vi "Dashboard Main.vi"() -> ()   [LabVIEW 2015]
uses:
  <vilib>/Utility/miscctls.llb/LVRowAndColumnTypeDef.ctl
  <vilib>/event_ctls.llb/eventvkey.ctl
  <vilib>/Rock Robotics/WPI/Dashboard/WPI_DashboardLogging Global.vi
  <vilib>/Rock Robotics/Network Tables/NT Write Boolean.vi
  <vilib>/Rock Robotics/Network Tables/NT Read Boolean.vi
  <vilib>/Utility/config.llb/Write Key (String).vi
  <vilib>/Utility/config.llb/Write Key (I32).vi
  <vilib>/Utility/config.llb/NI_LVConfig.lvlib
  <vilib>/vision/NI_Vision_Development_Module.lvlib
panel:
  out "Best Box":dbl[](array[numeric])
  in  "TCP":refnum<k5>
  in  "Rec Mode":enum32{"Stop", "Record", "Playback"}(radio)
  in  "Vision":u16(ring) items=["Camera Off", "USB Camera SW", "USB Camera HW", "IP Camera"]
  out "Camera IP":string
  out "Image Message":string="Timeout in Camera Communications"
  in  "Dashboard Tab":T1(tab)
  out "R Abv 60000":bool
  out "L Abv 60000":bool
  out "On Goal":bool
  out "Angler":dbl
  out "Right Shooter":dbl
  out "Left Shooter":dbl
  out "Right Ready":bool
  out "Left Ready":bool
  out "NT Connection":bool
  in  "Camera Settings":T2={"Frame Rate"=30, "Compression"=30, "Size"=1} {"Frame Rate" scale=1.0..30.0; "Size" items=["640x480", "320x240", "160x120"]}
  out "Gyro":cluster{dbl, dbl}(knob) scale=0.0..360.0
  out "Mode":T3(ring)=enum."Auto Disabled"
  in  "DB Camera Config":bool
  out "fps":dbl format="%#.1g"
  out "Mbps":dbl format="%#.1g"
  out "Mbps LED":bool
  out "View":bool
  in  "DB/String 9":string
  in  "DB/String 8":string
  in  "DB/String 7":string
  in  "DB/String 6":string
  in  "DB/String 5":string
  in  "DB/String 4":string
  in  "DB/String 3":string
  in  "DB/String 2":string
  in  "DB/String 1":string
  in  "DB/String 0":string
  in  "DB/Slider 0":dbl(slide) scale=0.0..5.0
  in  "DB/Slider 1":dbl(slide) scale=0.0..5.0
  in  "DB/Slider 2":dbl(slide) scale=0.0..5.0
  in  "DB/Slider 3":dbl(slide) scale=0.0..5.0
  out "DB/LED 3":bool
  out "DB/LED 2":bool
  out "DB/LED 1":bool
  out "DB/LED 0":bool
  in  "DB/Button 3":bool
  in  "DB/Button 2":bool
  in  "DB/Button 1":bool
  in  "DB/Button 0":bool caption="New Name"
  in  "Debug Camera":bool
  in  "Starting Direction":enum32{"Radio Selection 1", "Radio Selection 2"}(radio)
  in  "Defense to Cross":u16(ring) items=["Low Bar", "Moat", "Ramparts", "Rock Wall", "Rough Terrain", "Cheval", "Portculis"]
  in  "Starting Position":u16(ring) items=["1", "2", "3", "4", "5", "Spy"]
  in  "Autonomous Mode":u16(ring) items=["Do Nothing", "Drive to OW", "Drive through OW", "Shoot"]
  in  "Test Slider":dbl(slide) scale=0.0..100.0 scale format="%#_3g"
  in  "On/Off":bool caption="Solenoid"
  in  "Test Name":u16(ring) items=["Select the test to run..."]
  in  "Test Tree":string(tree)
  in  "Motor":cluster{"Value":dbl, "Enable":bool} {"Value" scale=-1.0..1.0 scale format="%#_3g"}
  out "Progress":T4 {"Test Progress" scale=0.0..100.0}
  in  "Rev/Fwd":cluster{"Forward":bool, "Reverse":bool}
  in  "Test Ring":u16(ring) items=["Monochrome", "Color"]
  out "Cmd Status":string
  in  "Execute Command":bool
  in  "Command Params":string[][](table)
  in  "Command Selection":i32(listbox)
  in  "CheckList":i32(listbox)
  out "Tree":string(tree)
  out "Camera Image":T5(plugin-control)
  out "Background":bool
  in  "Select Auto":string(combo)
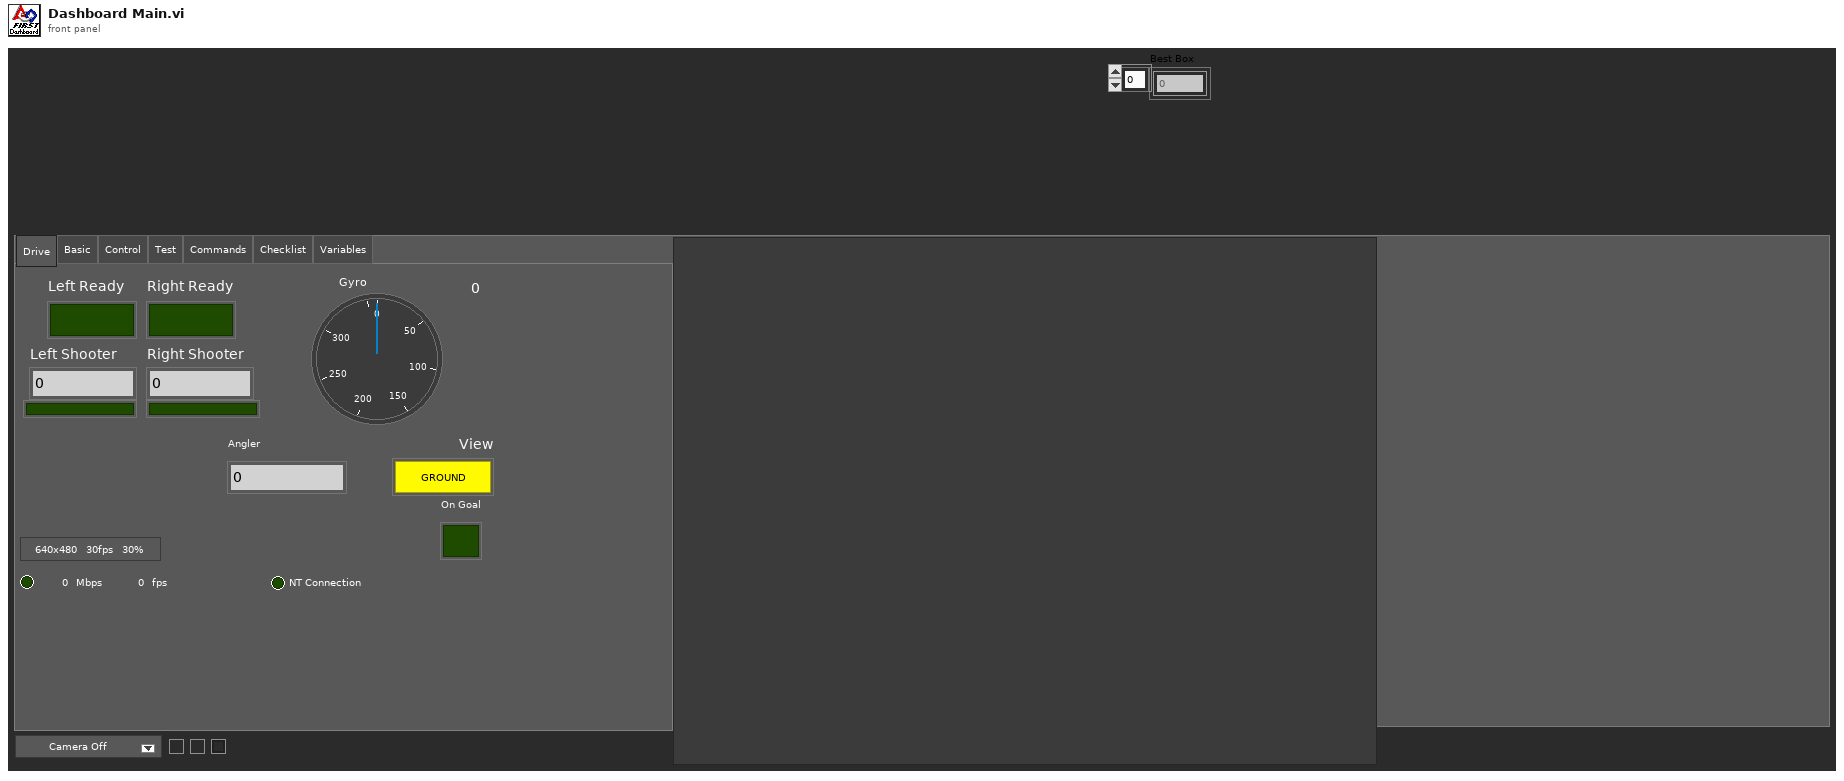
[diagram p1: front panel]
types:
  T1 = enum32{"Drive", "Basic", "Control", "Test", "Commands", "Checklist", "Variables"}
  T2 = cluster{"Frame Rate":i32, "Compression":i32, "Size":u16}
  T3 = enum8{"Tele-Op Disabled", "Tele-Op Enabled", "Auto Disabled", "Auto Enabled", "Test Disabled", "Test Enabled", "Disconnected", "No Code", "E-Stop"}
  T4 = cluster{"Test Progress":u8, "Test Progress Text":string}
  T5 = typedef "IMAQ Image.ctl" = refnum<image>
  T6 = cluster{"IDs":cluster{"RPC field ID":u16, "Unique ID":u16}, "String":string}
  T7 = enum32{"Drive", "Basic", "Custom", "Test", "Checklist", "Variables"}
  T8 = typedef "Image Type" = u32
  T9 = cluster{"Camera Image":refnum<vi>, "Dashboard Tab":refnum<vi>, "Background":refnum<vi>, "Vision":refnum<vi>, "Rec Mode":refnum<vi>, "Test Slider":refnum<vi>, "On/Off ":refnum<vi>, "Test Ring":refnum<vi>, "Rev/Fwd":refnum<vi>, "Test Name":refnum<vi>, "Motor":refnum<vi>, "Progress":refnum<vi>, "CheckList":refnum<vi>, "Tree":refnum<vi>, "Test Tree":refnum<vi>, "Command Params":refnum<vi>, "Command Selection":refnum<vi>, "Execute Command":refnum<vi>, "Cmd Status":refnum<vi>}
  T10 = cluster{"Error Strings":string, "Disable Counts":cluster{u16, u16}, "Rail Faults":cluster{u16, u16, u16}, "Robot IP":string, "DB Mode":u8, "Event Info":cluster{"Name":string, "Type":u8, "Number":u16, "Replay":u8}, "Camera Addr":string}
  T11 = cluster{"Storage":cluster{"Disk Free":u64, "RAM Block":u32, "RAM free":u32}, "CPU Utilization":cluster{"CPU % ISR":sgl, "CPU % Time Crit":sgl, "CPU % Timed Str":sgl, "CPU % High":sgl, "CPU % Above":sgl, "CPU % Normal":sgl, "CPU % Low":sgl}, "CAN":cluster{"% Bus Utilization":sgl, "Bus Off Cnt":u32, "TX_FIFO Full Cnt":u32, "Receive Error Cnt":u8, "Transmit Error Cnt":u8}, "HID":cluster{"HID Outputs":u32, "Rumble Low":u16, "Rumble High":u16}[]}
  T12 = cluster{"Status bits":cluster{"Test Mode":bool, "Autonomous":bool, "Enabled":bool, "Code Start":bool, "Brownout":bool, "Reserved 2":bool, "Reserved 3":bool, "E-Stop":bool}, "Code Trace":cluster{"Disabled":bool, "TeleOp":bool, "Auto":bool, "Test":bool}, "Controller Type":enum16{"unknown", "cRIO", "roboRio"}, "Code?":enum16{"unknown", "noCode", "code"}, "Battery V":dbl}
  T13 = cluster{"Control Bits":cluster{"TestMode":bool, "Autonomous":bool, "Enabled":bool, "FMS Present":bool, bool, bool, bool, "E-Stop":bool}, "Team Station ":u8, "Countdown":sgl, "Joystick Values":cluster{"Axes":dbl[], "Buttons":bool[], "POVs":i16[]}[]}
  T14 = typedef "NI_LVConfig.lvlib/Config Data RefNum.ctl" = refnum<k1>
  T15 = cluster{"Operation":enum16{"Update", "Clear"}, "Color Box":u32}[]
  T16 = typedef "eventvkey.ctl" = enum16{"ASCII", "Enter", "Return", "Shift", "Ctrl", "Alt", "Cmd", "Opt", "Caps", "NumLock", "Clear", "Break", "Up", "Down", "Left", "Right", "Insert", "Delete", "Home", "End", "PageUp", "PageDown", "Escape", "Help", "Pause", "ScrollLock", "F1", "F2", "F3", "F4", "F5", "F6", "F7", "F8", "F9", "F10", "F11", "F12", "F13", "F14", "F15", "F16", "F17", "F18", "F19", "F20", "F21", "F22", "F23", "F24", "Play", "VolumeUp", "VolumeDown", "Mute", "Two Byte Char"}
  T17 = cluster{"Image Size":bool, "Image Type":bool, "Pixel Value":bool, "ROI Information":bool, "Zoom Factor":bool}
  T18 = enum8{"Enabled", "Disabled", "Disabled and Grayed Out"}
  T19 = cluster{"Operation":enum16{"Update", "Clear"}, "Color Box":u32}
  T20 = typedef "LVRowAndColumnTypeDef.ctl" = cluster{"Row":i32, "Column":i32}
  T21 = cluster{"Shift":bool, "Ctrl":bool, "Alt":bool, "Cmd":bool, "Opt":bool}
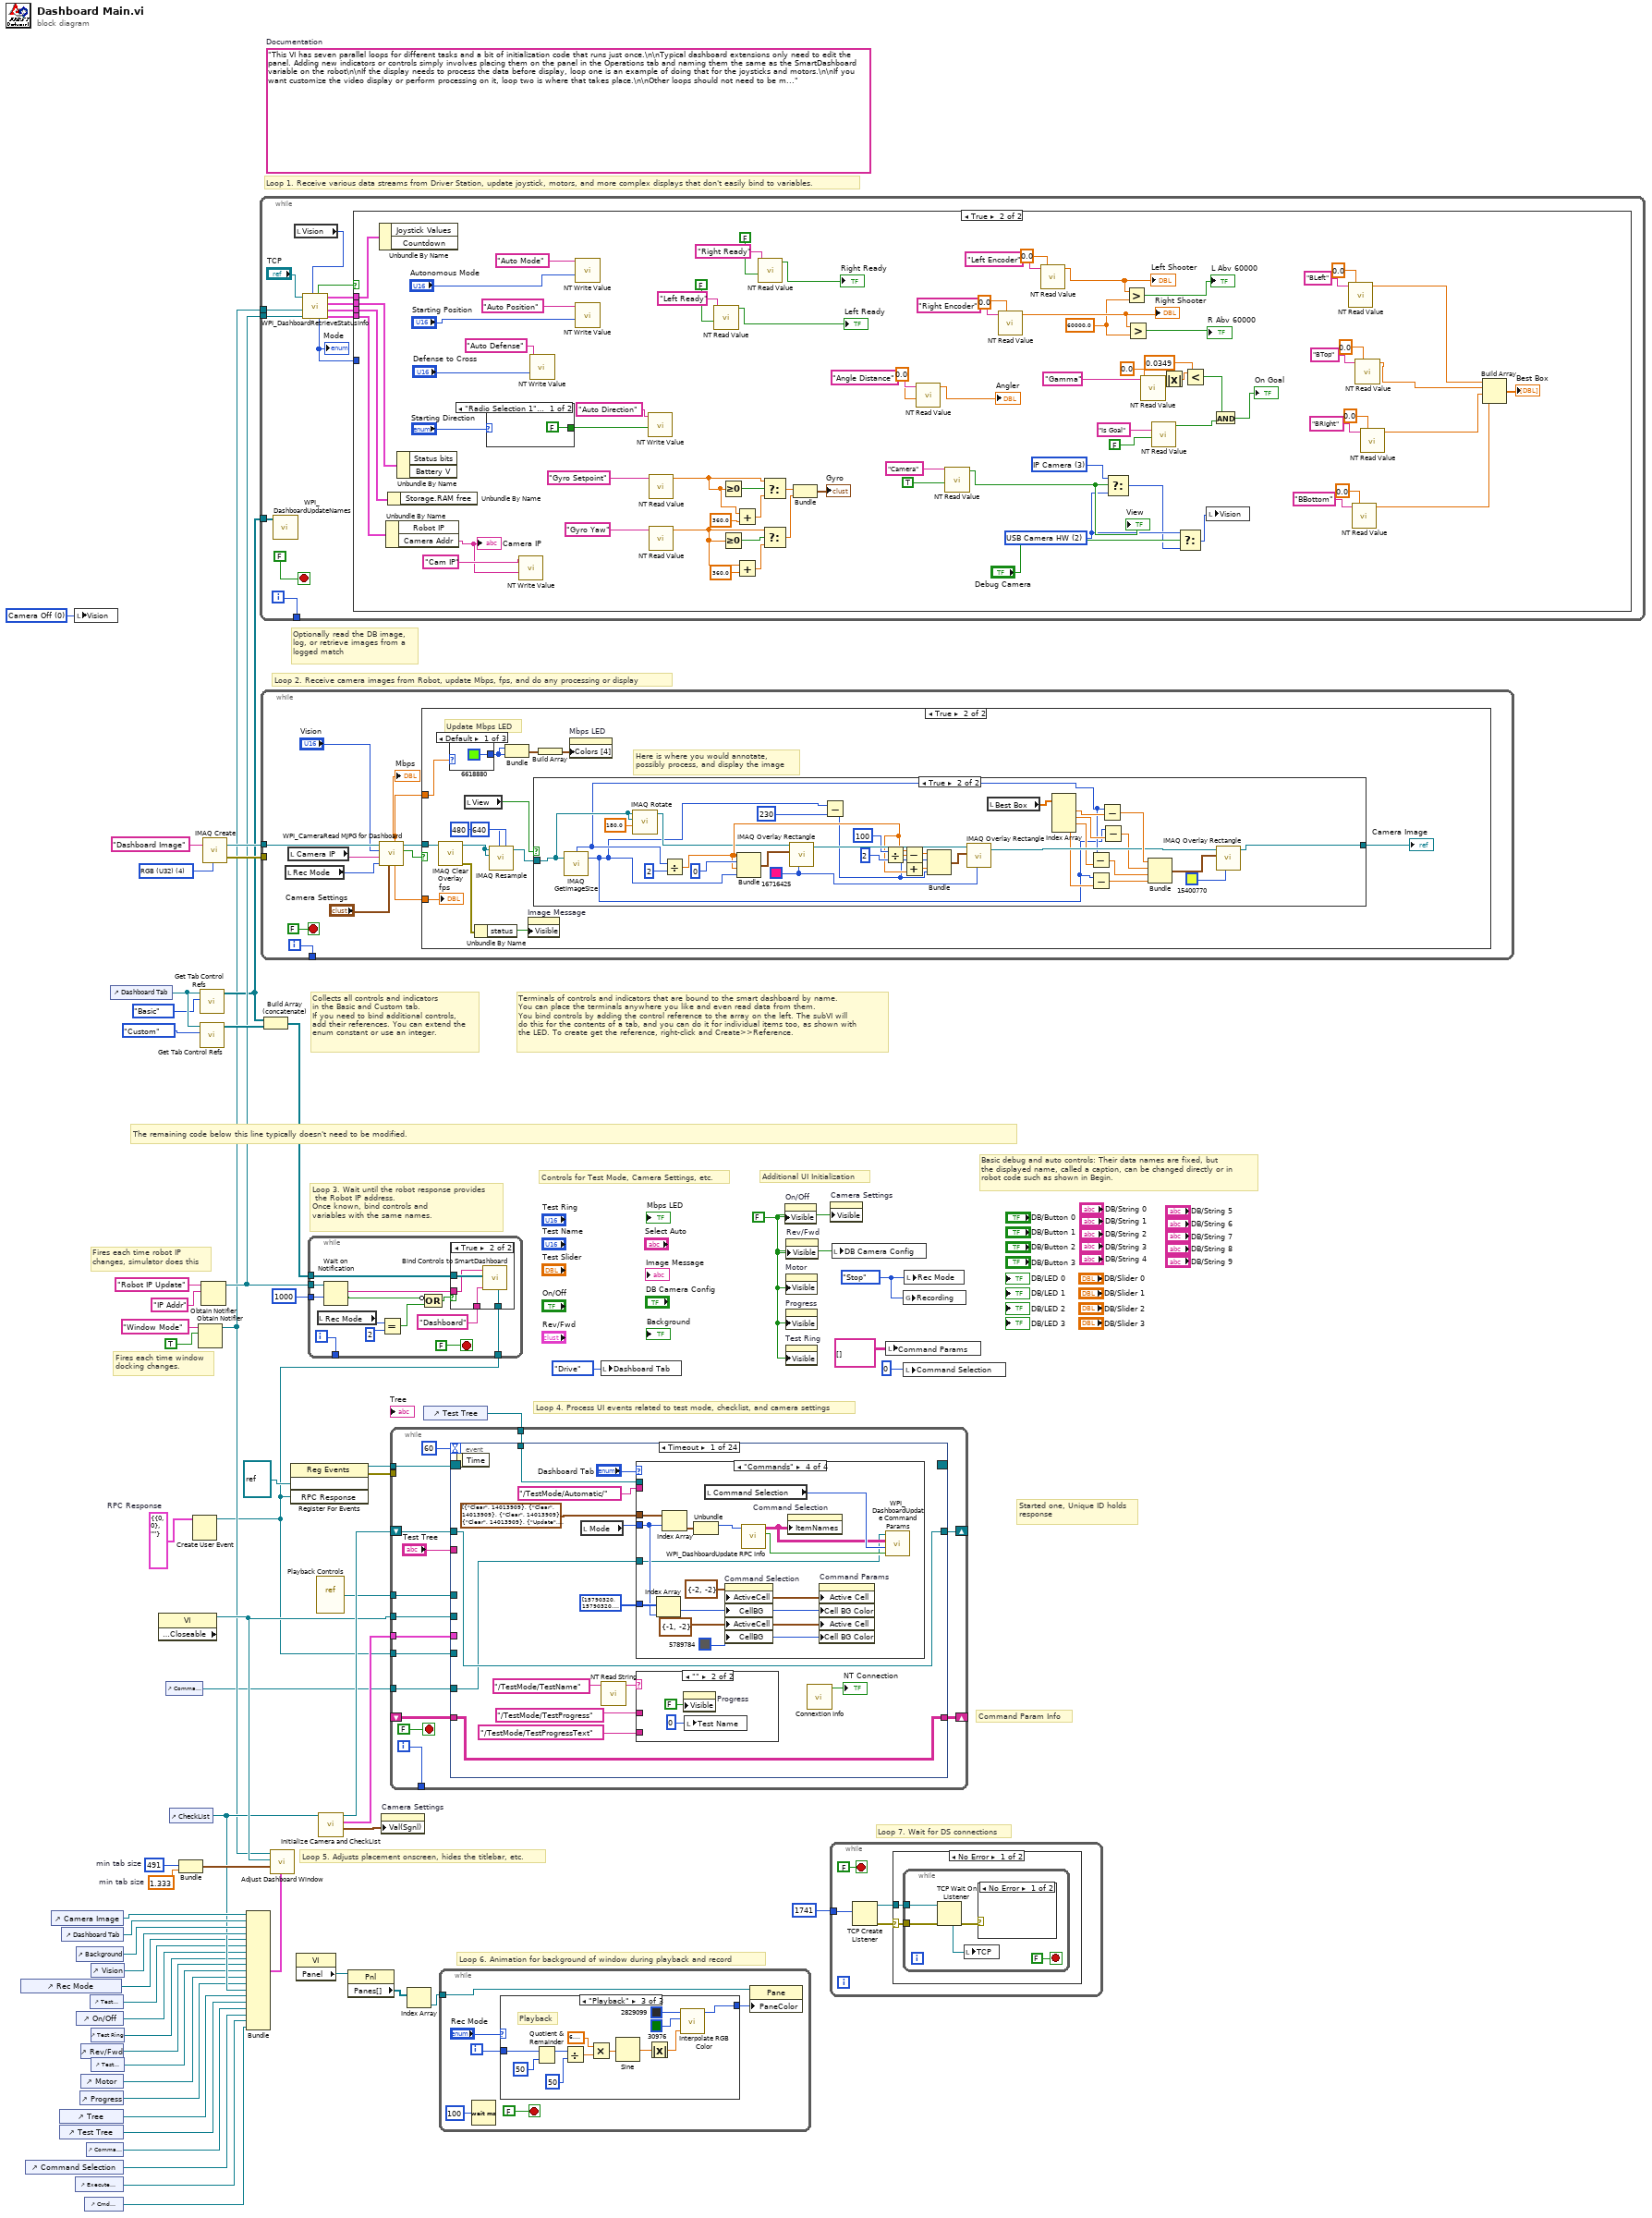
[diagram p0: block diagram]
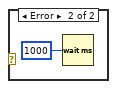
[diagram p2: hidden frame]
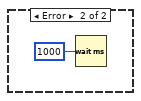
[diagram p3: hidden frame]
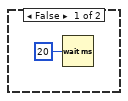
[diagram p4: hidden frame]
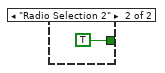
[diagram p5: hidden frame]
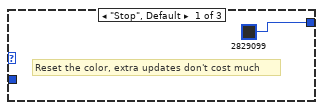
[diagram p6: hidden frame]
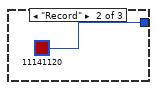
[diagram p7: hidden frame]
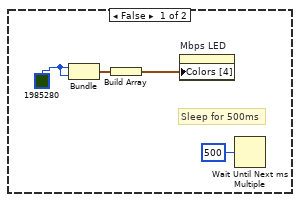
[diagram p9: hidden frame]
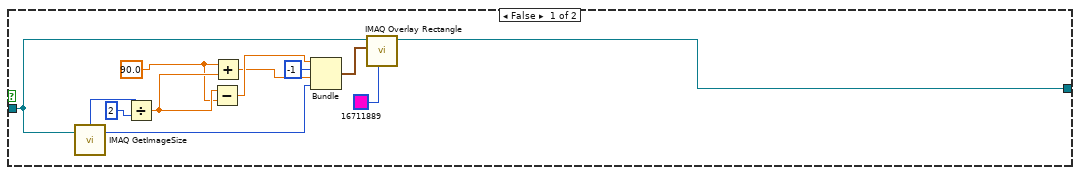
[diagram p10: hidden frame]
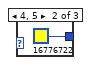
[diagram p11: hidden frame]
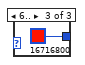
[diagram p12: hidden frame]
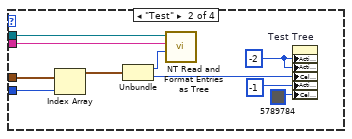
[diagram p14: hidden frame]
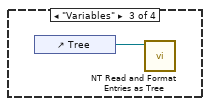
[diagram p15: hidden frame]
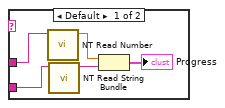
[diagram p16: hidden frame]
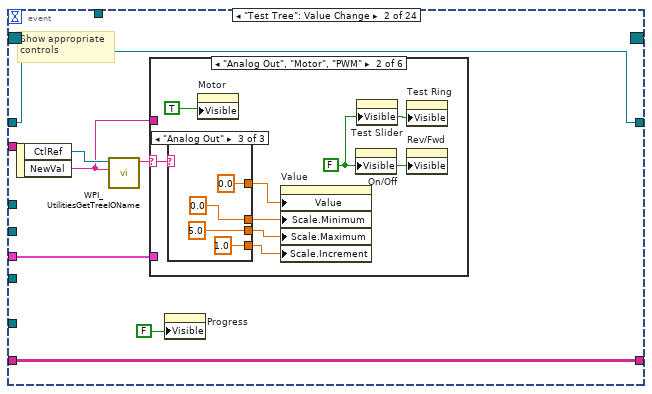
[diagram p17: hidden frame]
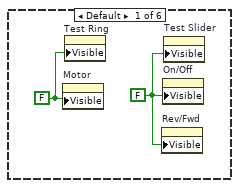
[diagram p18: hidden frame]
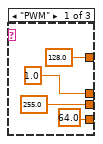
[diagram p19: hidden frame]
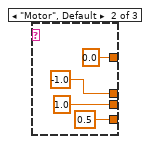
[diagram p20: hidden frame]
diagram:
  w1 = u16 0 items=["Camera Off", "USB Camera SW", "USB Camera HW", "IP Camera"] ("Vision")
  w9 = T6 {"IDs"={"RPC field ID"=0, "Unique ID"=0}, "String"=""}  # RPC Response
  w34 = 491  # min tab size
  w33 = 1.333  # min tab size
  w42 = enum32{"Stop", "Record", "Playback"}."Stop" ("Rec Mode")
  w16 = FALSE ("Visible")
  (unwired) "This VI has seven parallel loops for different tasks and a bit of initialization code that runs just once.\n\nTypical dashboard extensions only need to edit the panel. Adding new indicators or controls simply involves placing them on the panel in the Operations tab and naming them the same as the SmartDashboard variable on the robot\n\nIf the display needs to process the data before display, loop one is an example of doing that for the joysticks and motors.\n\nIf you want customize the video display or perform processing on it, loop two is where that takes place.\n\nOther loops should not need to be modified. They are pretty standard, and document the task they perform."  # Documentation
  w62 = T8 4 items=["Grayscale (U8)", "Grayscale (I16)", "Grayscale (SGL)", "Complex (CSG)", "RGB (U32)", "HSL (U32)", "RGB (U64)"] ("Image Type")
  # "Optionally read the DB image,\nlog, or retrieve images from a\nlogged match"
  # "Command Param Info"
  # "Started one, Unique ID holds\nresponse"
  # "Loop 7. Wait for DS connections"
  # "Basic debug and auto controls: Their data names are fixed, but\nthe displayed name, called a caption, can be changed directly or in\nrobot code such as shown in Begin."
  # "Controls for Test Mode, Camera Settings, etc."
  # "Additional UI Initialization"
  # "Loop 6. Animation for background of window during playback and record"
  # "Fires each time robot IP\nchanges, simulator does this"
  # "Fires each time window\ndocking changes."
  # "Collects all controls and indicators\nin the Basic and Custom tab.\nIf you need to bind additional controls,\nadd their references. You can extend the\nenum constant or use an integer."
  # "The remaining code below this line typically doesn't need to be modified."
  # "Loop 4. Process UI events related to test mode, checklist, and camera settings"
  # "Terminals of controls and indicators that are bound to the smart dashboard by name.\nYou can place the terminals anywhere you like and even read data from them.\nYou bind controls by adding the control reference to the array on the left. The subVI will\ndo this for the contents of a tab, and you can do it for individual items too, as shown with\nthe LED. To create get the reference, right-click and Create>>Reference."
  # "Loop 3. Wait until the robot response provides\n the Robot IP address.\nOnce known, bind controls and\nvariables with the same names."
  # "Loop 5. Adjusts placement onscreen, hides the titlebar, etc."
  # "Loop 1. Receive various data streams from Driver Station, update joystick, motors, and more complex displays that don't easily bind to variables."
  # "Loop 2. Receive camera images from Robot, update Mbps, fps, and do any processing or display"
  n1 = control-ref of="Rec Mode"() -> (w22:refnum<vi>)
  n2 = control-ref of="Command Selection"() -> (w8:refnum<vi>)
  n3 = control-ref of="Camera Image"() -> (w37:refnum<vi>)
  n4 = control-ref of="Tree"() -> (w26:refnum<vi>)
  n5 = control-ref of="Test Tree"() -> (w25:refnum<vi>)
  n6 = control-ref of="Dashboard Tab"() -> (w36:refnum<vi>)
  n7 = local write "Vision"(w1) -> ()
  n8 = control-ref of="Execute Command"() -> (w10:refnum<vi>)
  n9 = control-ref of="Background"() -> (w31:refnum<vi>)
  n10 = control-ref of="On/Off"() -> (w20:refnum<vi>)
  n11 = control-ref of="Progress"() -> (w17:refnum<vi>)
  n12 = control-ref of="Rev/Fwd"() -> (w18:refnum<vi>)
  n13 = control-ref of="Motor"() -> (w23:refnum<vi>)
  n14 = control-ref of="Cmd Status"() -> (w4:refnum<vi>)
  n15 = control-ref of="Command Params"() -> (w11:refnum<vi>)
  n16 = control-ref of="Test Slider"() -> (w21:refnum<vi>)
  n17 = control-ref of="Vision"() -> (w35:refnum<vi>)
  n18 = control-ref of="Test Ring"() -> (w19:refnum<vi>)
  n19 = control-ref of="Test Name"() -> (w24:refnum<vi>)
  n20 = control-ref of="Dashboard Tab"() -> (w40:refnum<vi>)
  n21 = property class="VI" props=["Front Panel.Closeable"]() -> (reference out=w41:refnum<vi>)  [unwired: 2 in, 2 out]
  n22 = control-ref of="Command Params"() -> (w3:refnum<vi>)
  n23 = control-ref of="CheckList"() -> (w27:refnum<vi>)
  n24 = Bundle("min tab size"=w34, "min tab size"=w33) -> (w32:cluster{"min tab size":i32, "min tab size":dbl})  [unwired: 1 in]
  n25 = Create User Event(user event datatype=w9) -> (user event=w5:refnum<user-event>)  [unwired: 1 in, 1 out]
  n26 = Obtain Notifier(name (unnamed)="Window Mode", notification data type=TRUE) -> (notifier out=w13:refnum<notifier>)  [unwired: 2 in, 2 out]
  n27 = call <vilib>:"Get Tab Control Refs.vi"("Page Index"=T7."Basic" ("Dashboard Tab"), "TabControl in"=w40) -> ("ControlsOnPage"=w14:refnum<vi>[])  [unwired: 9 in]
  n28 = call <vilib>:"Get Tab Control Refs.vi"("Page Index"=T7."Custom" ("Dashboard Tab"), "TabControl in"=w40) -> ("ControlsOnPage"=w39:refnum<vi>[])  [unwired: 9 in]
  n29 = Obtain Notifier(name (unnamed)="Robot IP Update", notification data type="IP Addr" ("name (unnamed)")) -> (notifier out=w15:refnum<notifier>)  [unwired: 2 in, 2 out]
  n30 = call "IMAQ Create"("Image Name"="Dashboard Image", "Image Type"=w62) -> ("New Image"=w60:T5, "error out"=w59:errorcluster)  [unwired: 2 in, 1 out]
  n31 = Bundle("Camera Image"=w37, "Dashboard Tab"=w36, "Background"=w31, "Vision"=w35, "Rec Mode"=w22, "Test Slider"=w21, "On/Off"=w20, "Test Ring"=w19, "Rev/Fwd"=w18, "Test Name"=w24, "Motor"=w23, "Progress"=w17, "CheckList"=w27, "Tree"=w26, "Test Tree"=w25, "Command Params"=w11, "Command Selection"=w8, "Execute Command"=w10, "Cmd Status"=w4) -> (w28:T9)  [unwired: 1 in]
  n32 = while {
    tunnel: [w74] -> _
    tunnel: w15 -> [w68]
    tunnel: w14 -> [w67]
    tunnel: w13 -> [w64]
    i -> [w74]
    stop <- FALSE stop-if-true
    n33 = call <vilib>:"WPI_DashboardUpdateNames.vi"("Controls on Tab"=w67) -> ()  [unwired: 11 in]
    n34 = local read "Vision"() -> (w63:u16)
    n35 = call <vilib>:"WPI_DashboardRetrieveStatusInfo.vi"("Vision"=w63, "Binding Refnum"=w68, "Window Mode Notifier"=w64, "TCP Cnx"="TCP") -> ("Power and Errors"=w69:T10, "Robot Metrics"=w72:T11, "Status Info"=w73:T12, "Control Info"=w70:T13, "Robot Mode"=w66:T3, "Process?"=w71:bool)  [unwired: 2 in]
    "Mode" <- w66
    n36 = case shown="True" w71 {
      tunnel: w73 -> [_ w153]
      tunnel: w72 -> [_ w152]
      tunnel: w70 -> [_ w151]
      tunnel: w69 -> [_ w150]
      tunnel: w66 -> [_ _]
      frame False {
        n37 = Wait (ms)(milliseconds to wait=u32 20) -> ()  [unwired: 1 out]
      }
      frame True {
        w105 = 60000.0 ("y")
        w79 = u16 2 items=["Camera Off", "USB Camera SW", "USB Camera HW", "IP Camera"] ("Camera Mode")
        w82 = u16 3 items=["Camera Off", "USB Camera SW", "USB Camera HW", "IP Camera"] ("Camera Mode")
        n38 = Unbundle By Name(w151) -> ()  [unwired: 2 out]
        n39 = Unbundle By Name(w150) -> ("Camera Addr"=w101:string)  [unwired: 1 out]
        "Camera IP" <- w101
        n40 = Unbundle By Name(w152) -> ()  [unwired: 1 out]
        n41 = Unbundle By Name(w153) -> ()  [unwired: 2 out]
        n42 = case shown="\"Radio Selection 1\", Default" "Starting Direction" {
          tunnel: [FALSE TRUE] -> w148
          frame "Radio Selection 1", Default {
          }
          frame "Radio Selection 2" {
          }
        }
        n43 = call-poly <vilib>:"NT Write Value.vi"("String"=w101, "Name"="Cam IP") -> ()  [unwired: 9 in, 1 out]
        n44 = call-poly <vilib>:"NT Write Value.vi"("Numeric"="Defense to Cross", "Name"="Auto Defense") -> ()  [unwired: 9 in, 1 out]
        n45 = call-poly <vilib>:"NT Write Value.vi"("Numeric"="Autonomous Mode", "Name"="Auto Mode") -> ()  [unwired: 9 in, 1 out]
        n46 = call-poly <vilib>:"NT Write Value.vi"("Numeric"="Starting Position", "Name"="Auto Position") -> ()  [unwired: 9 in, 1 out]
        n47 = call-poly <vilib>:"NT Write Value.vi"("Boolean"=w148, "Name"="Auto Direction") -> ()  [unwired: 9 in, 1 out]
        n48 = call-poly <vilib>:"NT Read Value.vi"("Name"="Gyro Setpoint") -> ("Numeric"=w118:dbl)  [unwired: 9 in, 1 out]
        n49 = call-poly <vilib>:"NT Read Value.vi"("Name"="Gyro Yaw") -> ("Numeric"=w126:dbl)  [unwired: 9 in, 1 out]
        n50 = call-poly <vilib>:"NT Read Value.vi"("Default Value"=FALSE, "Name"="Left Ready") -> ("Boolean"=→"Left Ready":bool)  [unwired: 8 in, 1 out]
        n51 = Greater Or Equal To 0?(x=w118) -> (x >= 0?=w124:bool)
        n52 = Greater Or Equal To 0?(x=w126) -> (x >= 0?=w128:bool)
        n53 = Add(x=w118, y=360.0) -> (x+y=w123:dbl)
        n54 = Add(x=w126, y=360.0) -> (x+y=w127:dbl)
        n55 = call-poly <vilib>:"NT Read Value.vi"("Default Value"=FALSE, "Name"="Right Ready") -> ("Boolean"=→"Right Ready":bool)  [unwired: 8 in, 1 out]
        n56 = Select(t=w118, s=w124, f=w123) -> (s? t:f=w121:dbl)
        n57 = Select(t=w126, s=w128, f=w127) -> (s? t:f=w120:dbl)
        n58 = Bundle("Numeric"=w121, "Numeric"=w120) -> (→"Gyro":cluster{"Numeric":dbl, "Numeric":dbl})  [unwired: 1 in]
        n59 = call-poly <vilib>:"NT Read Value.vi"("Default Value"=0.0, "Name"="Angle Distance") -> ("Numeric"=→"Angler":dbl)  [unwired: 8 in, 1 out]
        n60 = call-poly <vilib>:"NT Read Value.vi"("Default Value"=TRUE, "Name"="Camera") -> ("Boolean"=w81:bool)  [unwired: 8 in, 1 out]
        "View" <- w81
        n61 = call-poly <vilib>:"NT Read Value.vi"("Default Value"=0.0, "Name"="Right Encoder") -> ("Numeric"=w106:dbl)  [unwired: 8 in, 1 out]
        "Right Shooter" <- w106
        n62 = call-poly <vilib>:"NT Read Value.vi"("Default Value"=0.0, "Name"="Left Encoder") -> ("Numeric"=w107:dbl)  [unwired: 8 in, 1 out]
        "Left Shooter" <- w107
        n63 = Select(t=w82, s=w81, f=w79) -> (s? t:f=w78:u16)
        n64 = Greater?(x=w107, y=w105) -> (0:→"L Abv 60000":bool)
        n65 = Greater?(x=w106, y=w105) -> (0:→"R Abv 60000":bool)
        n66 = call-poly <vilib>:"NT Read Value.vi"("Default Value"=0.0, "Name"="Gamma") -> ("Numeric"=w112:dbl)  [unwired: 8 in, 1 out]
        n67 = call-poly <vilib>:"NT Read Value.vi"("Default Value"=FALSE, "Name"="Is Goal") -> ("Boolean"=w96:bool)  [unwired: 8 in, 1 out]
        n68 = Absolute Value(x=w112) -> (abs(x)=w111:dbl)
        n69 = Select(t=w79, s="Debug Camera", f=w78) -> (s? t:f=w77:u16)
        n70 = Less?(x=w111, y=0.0349) -> (x < y?=w98:bool)
        n71 = local write "Vision"(w77) -> ()
        n72 = And(x=w98, y=w96) -> (x .and. y?=→"On Goal":bool)
        n73 = call-poly <vilib>:"NT Read Value.vi"("Default Value"=0.0, "Name"="BLeft") -> ("Numeric"=w87:dbl)  [unwired: 8 in, 1 out]
        n74 = call-poly <vilib>:"NT Read Value.vi"("Default Value"=0.0, "Name"="BBottom") -> ("Numeric"=w84:dbl)  [unwired: 8 in, 1 out]
        n75 = call-poly <vilib>:"NT Read Value.vi"("Default Value"=0.0, "Name"="BTop") -> ("Numeric"=w86:dbl)  [unwired: 8 in, 1 out]
        n76 = call-poly <vilib>:"NT Read Value.vi"("Default Value"=0.0, "Name"="BRight") -> ("Numeric"=w85:dbl)  [unwired: 8 in, 1 out]
        n77 = Build Array(w87, w86, w85, w84) -> (→"Best Box":dbl[])
      }
    }
  }
  n78 = while {
    tunnel: w60 -> [w164]
    tunnel: w59 -> [_]
    tunnel: [w165] -> _
    i -> [w165]
    stop <- FALSE stop-if-true
    n79 = local read "Rec Mode"() -> (w159:enum32{"Stop", "Record", "Playback"})
    n80 = local read "Camera IP"() -> (w158:string)
    n81 = call <vilib>:"WPI_CameraRead MJPG for Dashboard.vi"("Camera Settings"="Camera Settings", "Rec Mode"=w159, "Camera IP"=w158, "Camera Mode"="Vision", "Refnum in"=w164) -> ("Active"=w162:bool, "Refnum out"=w163:T5, "FPS"=w161:dbl, "Bandwidth (Mbps)"=w157:dbl)  [unwired: 3 in]
    "Mbps" <- w157
    n82 = case shown="True" w162 {
      tunnel: w163 -> [_ w179]
      tunnel: w157 -> [_ w178]
      tunnel: w161 -> [_ w177]
      frame False {
        w167 = u32 1985280 ("Color Box")
        # "Sleep for 500ms"
        n83 = Bundle("Color Box"=w167, "Color Box"=w167) -> (w169:cluster{"Color Box":u32, "Color Box":u32})  [unwired: 1 out]
        n84 = Build Array(w169) -> (w168:cluster{"Color Box":u32, "Color Box":u32}[])
        n85 = property on="Mbps LED" class="Bool (strict)"("Colors [4]"=w168) -> ()  [unwired: 2 in, 2 out]
        n86 = Wait Until Next ms Multiple(millisecond multiple=u32 500) -> ()  [unwired: 1 out]
      }
      frame True {
        # "Here is where you would annotate,\npossibly process, and display the image"
        # "Update Mbps LED"
        n87 = call "IMAQ Clear Overlay"("Image"=w179) -> ("error out"=w183:errorcluster, "Image Out"=w173:T5)  [unwired: 2 in, 7 out]
        n88 = case shown="Default" w178 {
          tunnel: [u32 6618880 ("Color Box") u32 16776722 ("Color Box") u32 16716800 ("Color Box")] -> w180
          frame Default {
          }
          frame 4, 5 {
          }
          frame 6.. {
          }
        }
        n89 = local read "View"() -> (w175:bool)
        n90 = Unbundle By Name(w183) -> ("status"=w184:bool)
        n91 = call "IMAQ Resample"("X Resolution"=640, "Y Resolution"=480, "Image Dst"=w173, "Image Src"=w173) -> ("Image Dst Out"=w174:T5)  [unwired: 6 in, 1 out]
        n92 = Bundle("Color Box"=w180, "Color Box"=w180) -> (w182:cluster{"Color Box":u32, "Color Box":u32})  [unwired: 1 out]
        n93 = property on="Image Message" class="Str"("Visible"=w184) -> ()  [unwired: 2 in, 2 out]
        n94 = case shown="True" w175 {
          tunnel: [w195 w207] -> w176
          tunnel: w174 -> [w196 w215]
          frame False {
            w188 = 90.0
            n95 = call "IMAQ GetImageSize"("Image"=w196) -> ("Y Resolution"=w193:i32, "X Resolution"=w190:i32)  [unwired: 3 in, 1 out]
            n96 = Divide(x=w190, y=2) -> (x/y=w189:dbl)
            n97 = Subtract(x=w189, y=w188) -> (x-y=w187:dbl)
            n98 = Add(x=w188, y=w189) -> (x+y=w186:dbl)
            n99 = Bundle(w187, -1, w186, "Y Resolution"=w193) -> (w194:cluster{dbl, i32, dbl, "Y Resolution":i32})  [unwired: 1 in]
            n100 = call "IMAQ Overlay Rectangle"("Color"=u32 16711889, "Rectangle"=w194, "Image"=w196) -> ("Image Out"=w195:T5)  [unwired: 7 in, 1 out]
          }
          frame True {
            w217 = u32 16716425 ("Color")
            n101 = call "IMAQ GetImageSize"("Image"=w215) -> ("Y Resolution"=w199:i32, "X Resolution"=w200:i32)  [unwired: 3 in, 1 out]
            n102 = call "IMAQ Rotate"("Angle (degrees)"=sgl 180.0, "Image Dst"=w215, "Image Src"=w215) -> ("Image Dst Out"=w214:T5)  [unwired: 7 in, 1 out]
            n103 = Divide(x=w200, y=2) -> (x/y=w219:dbl)
            n104 = Bundle(w219, 0, w219, "Y Resolution"=w199) -> (w228:cluster{dbl, i32, dbl, "Y Resolution":i32})  [unwired: 1 in]
            n105 = call "IMAQ Overlay Rectangle"("Color"=w217, "Rectangle"=w228, "Image"=w214) -> ("Image Out"=w225:T5)  [unwired: 7 in, 1 out]
            n106 = Subtract(x=w199, y=230) -> (x-y=w213:i32)
            n107 = Divide(x=100, y=2) -> (x/y=w220:dbl)
            n108 = Subtract(x=w219, y=w220) -> (x-y=w222:dbl)
            n109 = Add(x=w220, y=w219) -> (x+y=w221:dbl)
            n110 = Bundle(w222, w213, w221, w213) -> (w218:cluster{dbl, i32, dbl, i32})  [unwired: 1 in]
            n111 = call "IMAQ Overlay Rectangle"("Color"=w217, "Rectangle"=w218, "Image"=w225) -> ("Image Out"=w206:T5)  [unwired: 7 in, 1 out]
            n112 = local read "Best Box"() -> (w205:dbl[])
            n113 = Index Array(array=w205) -> (element #1=w204:dbl, element #2=w203:dbl, element #3=w201:dbl, element #4=w202:dbl)  [unwired: 4 in]
            n114 = Subtract(x=w200, y=w201) -> (x-y=w197:dbl)
            n115 = Subtract(x=w199, y=w202) -> (x-y=w209:dbl)
            n116 = Subtract(x=w200, y=w204) -> (x-y=w208:dbl)
            n117 = Subtract(x=w199, y=w203) -> (x-y=w198:dbl)
            n118 = Bundle(w208, w198, w197, w209) -> (w210:cluster{dbl, dbl, dbl, dbl})  [unwired: 1 in]
            n119 = call "IMAQ Overlay Rectangle"("Color"=u32 15400770, "Rectangle"=w210, "Image"=w206) -> ("Image Out"=w207:T5)  [unwired: 7 in, 1 out]
          }
        }
        "Camera Image" <- w176
        n120 = Build Array(w182) -> (w181:cluster{"Color Box":u32, "Color Box":u32}[])
        n121 = property on="Mbps LED" class="Bool (strict)"("Colors [4]"=w181) -> ()  [unwired: 2 in, 2 out]
        "fps" <- w177
      }
    }
  }
  n122 = Build Array (concatenate)(w14, w39) -> (w38:refnum<vi>[])
  n123 = call "Adjust Dashboard Window.vi"("Sizing Refnums"=w28, "Size Constraints"=w32, "VI"=w41, "WIn Mode"=w13) -> ()  [unwired: 8 in]
  n124 = register-events(refnum<vi> refnum, w5) -> (reference out=w46:refnum<event-registration>, error out=w45:errorcluster)  [unwired: 2 in]
  n125 = property class="VI"() -> ("Panel"=w49:refnum<vi>)  [unwired: 2 in, 2 out]
  n126 = while {
    tunnel: w38 -> [w244]
    tunnel: w15 -> [w242]
    tunnel: [w240] -> _
    tunnel: u32 1000 ("milliseconds to wait") -> [w239]
    tunnel: w5 -> [w232]
    i -> [w240]
    stop <- FALSE stop-if-true
    n127 = local read "Rec Mode"() -> (w235:enum32{"Stop", "Record", "Playback"})
    n128 = Wait on Notification(notifier=w242, timeout in ms (-1)=w239) -> (notification=w241:string, timed out?=w237:bool)  [unwired: 2 in, 2 out]
    n129 = Equal?(x=w235, y=u16 2 ("Rec Mode")) -> (x = y?=w236:bool)
    n130 = Compound Arithmetic op=OR(invert w237, w236) -> (w238:bool)
    n131 = case shown="True" w238 {
      tunnel: w244 -> [_ w248]
      tunnel: w241 -> [_ w247]
      tunnel: "Dashboard" -> [_ w246]
      tunnel: w232 -> [_ w245]
      frame False {
      }
      frame True {
        n132 = call <vilib>:"Bind Controls to SmartDashboard.vi"("RPC ref"=w245, "Client Name"=w246, "Bound Control Refs"=w248, "Server IP Address"=w247) -> ()  [unwired: 8 in]
      }
    }
  }
  n133 = vi-ref "Playback Controls.vi"() -> (w47:refnum<vi>)
  n134 = call "Initialize Camera and CheckList.vi"("ListBox in"=w27) -> ("Cluster"=w53:cluster{"value":i32, "value":i32, "index":i32}, "Array"=w54:cluster{string[]}[], "File Refnum"=w52:T14)  [unwired: 8 in]
  n135 = property class="Pnl"(reference=w49) -> ("Panes[]"=w50:refnum<vi>[])  [unwired: 1 in, 2 out]
  n136 = property on="Camera Settings" class="Clust (strict)"("Val(Sgnl)"=w53) -> ()  [unwired: 2 in, 2 out]
  n137 = Index Array(array=w50) -> (element=w48:refnum<vi>)  [unwired: 1 in]
  n138 = control-ref of="Test Tree"() -> (w51:refnum<vi>)
  n139 = while {
    tunnel: w54 -> [w260]
    shift-right: [w259] -> _
    shift-left: w52 -> [w258]
    tunnel: [w257] -> _
    tunnel: w51 -> [w256]
    tunnel: w47 -> [w255]
    tunnel: w46 -> [w254]
    tunnel: w45 -> [_]
    tunnel: w41 -> [w253]
    tunnel: w5 -> [w252]
    tunnel: w3 -> [w251]
    shift-right: [w250] -> _
    shift-left: _ -> [w249]
    i -> [w257]
    stop <- FALSE stop-if-true
    n140 = event shown="[0] Timeout" {
      selector: w254 -> [_ _ _ _ _ _ _ _ _ _ _ _ _ _ _ _ _ _ _ _ _ _ _ _]
      dyn-events: [_ _ _ _ _ _ _ _ _ _ _ _ _ _ _ _ _ _ w569 _ _ _ _ _] -> _
      timeout: u32 60 ("milliseconds to wait") -> [_ _ _ _ _ _ _ _ _ _ _ _ _ _ _ _ _ _ _ _ _ _ _ _]
      tunnel: w256 -> [w273 _ _ _ _ _ _ _ _ _ _ _ _ _ _ _ _ _ _ _ _ _ _ _]
      tunnel: "Test Tree" -> [_ _ _ _ _ _ _ _ _ _ _ _ _ w532 w541 w544 w549 w558 _ _ _ _ _ _]
      tunnel: w260 -> [_ w311 _ _ _ _ _ _ _ _ _ w494 w525 _ _ _ _ _ _ _ _ _ _ _]
      tunnel: [w270 w310 w414 w420 w430 w434 w440 w452 w460 w466 w479 w493 w518 w531 w539 w543 w548 w557 w571 w587 w589 w597 w608 w613] -> w259
      tunnel: w258 -> [w270 w310 w414 w420 w430 w434 w440 w452 w460 w466 w479 w492 w518 w531 w539 w543 w548 w557 w571 w587 w589 w597 w608 w613]
      tunnel: w255 -> [_ _ _ _ _ _ _ _ _ _ _ _ _ _ _ _ _ _ w572 _ w592 _ _ _]
      tunnel: w253 -> [_ _ _ _ _ _ _ _ _ _ _ _ _ _ _ _ _ _ w567 _ _ _ _ _]
      tunnel: w252 -> [_ _ _ _ _ _ _ _ _ _ _ _ _ _ _ _ _ _ w563 _ _ _ _ _]
      tunnel: w251 -> [w265 _ _ _ _ _ w438 _ _ _ _ _ _ _ _ _ _ _ _ _ _ _ _ _]
      tunnel: [w264 w309 w413 w419 w429 w435 w436 w446 w457 w465 w478 w491 w517 w530 w538 w542 w547 w556 w562 w585 w588 w593 w601 w614] -> w250
      tunnel: w249 -> [w264 w309 w413 w419 w429 w435 w436 _ _ w465 w478 w491 w517 w530 w538 w542 w547 w556 w562 w585 w588 w593 w601 w614]
      event Timeout {
        n141 = event-data() -> ()  [unwired: 1 in, 1 out]
        n142 = local read "Mode"() -> (w267:T3)
        n143 = call <vilib>:"NT Read String.vi"("Name"="/TestMode/TestName") -> ("String"=w276:string)  [unwired: 9 in, 1 out]
        n144 = case shown="\"Commands\"" "Dashboard Tab" {
          tunnel: w273 -> [_ w287 _ _]
          tunnel: "/TestMode/Automatic/" ("Name Pattern") -> [_ w286 _ _]
          tunnel: T15 [{"Operation"=enum."Clear", "Color Box"=14013909}, {"Operation"=enum."Clear", "Color Box"=14013909}, {"Operation"=enum."Clear", "Color Box"=14013909}, {"Operation"=enum."Clear", "Color Box"=14013909}, {"Operation"=enum."Update", "Color Box"=14013909}, {"Operation"=enum."Update", "Color Box"=16777215}, {"Operation"=enum."Clear", "Color Box"=14013909}, {"Operation"=enum."Clear", "Color Box"=14013909}, {"Operation"=enum."Clear", "Color Box"=14013909}] -> [_ w279 _ w296]
          tunnel: w267 -> [_ w278 _ w295]
          tunnel: u32[] [15790320, 15790320, 15790320, 15790320, 16777215, 16777215, 15790320, 15790320, 15790320] -> [_ _ _ w301]
          tunnel: w265 -> [_ _ _ w289]
          frame "Control", Default {
          }
          frame "Test" {
            w285 = -2 ("Active Item:Row Number")
            n145 = Index Array(array=w279, index=w278) -> (element=w280:T19)
            n146 = Unbundle(w280) -> ("Operation"=w281:enum16{"Update", "Clear"}, "Color Box"=w282:u32)
            n147 = call <vilib>:"NT Read and Format Entries as Tree.vi"("Operation"=w281, "Name Pattern"=w286, "Tree Refnum"=w287) -> ()  [unwired: 7 in, 2 out]
            n148 = property on="Test Tree" class="Tree (strict)"("Active Item Row Number"=w285, "ActiveColNum"=w285, "CellBG"=w282, "Active Item Row Number"=-1 ("Active Item:Row Number"), "CellBG"=u32 5789784 ("Color Box")) -> ()  [unwired: 2 in, 2 out]
          }
          frame "Variables" {
            n149 = control-ref of="Tree"() -> (w288:refnum<vi>)
            n150 = call <vilib>:"NT Read and Format Entries as Tree.vi"("Tree Refnum"=w288) -> ()  [unwired: 9 in, 2 out]
          }
          frame "Commands" {
            w297 = u32 5789784 ("Color Box")
            w298 = T20 {"Row"=-1, "Column"=-2} ("Active Cell:Active Cell")
            w300 = T20 {"Row"=-2, "Column"=-2} ("Active Cell:Active Cell")
            n151 = Index Array(array=w301, index=w295) -> (element=w299:u32)
            n152 = Index Array(array=w296, index=w295) -> (element=w294:T19)
            n153 = Unbundle(w294) -> ("Operation"=w293:enum16{"Update", "Clear"})  [unwired: 1 out]
            n154 = local read "Command Selection"() -> (w292:i32)
            n155 = property on="Command Selection" class="MCListbox (strict)"("ActiveCell"=w300, "CellBG"=w299, "ActiveCell"=w298, "CellBG"=w297) -> ()  [unwired: 2 in, 2 out]
            n156 = call <vilib>:"WPI_DashboardUpdate RPC Info.vi"("Operation"=w293) -> ("update"=w291:bool, "commands"=w290:string[][])  [unwired: 9 in]
            n157 = property on="Command Selection" class="MCListbox (strict)"("ItemNames"=w290) -> ()  [unwired: 2 in, 2 out]
            n158 = property on="Command Params" class="Tbl (strict)"("Active Cell"=w300, "Cell BG Color"=w299, "Active Cell"=w298, "Cell BG Color"=w297) -> ()  [unwired: 2 in, 2 out]
            n159 = call <vilib>:"WPI_DashboardUpdate Command Params.vi"("Update"=w291, "NewVal"=w292, "Commands"=w290, "Param Tbl"=w289) -> ()  [unwired: 7 in, 1 out]
          }
        }
        n160 = case shown="\"\"" w276 {
          tunnel: "/TestMode/TestProgress" ("Name") -> [w303 _]
          tunnel: "/TestMode/TestProgressText" ("Name") -> [w302 _]
          frame Default {
            n161 = call <vilib>:"NT Read Number.vi"("Name"=w303) -> ("Numeric"=w304:dbl)  [unwired: 9 in, 1 out]
            n162 = call <vilib>:"NT Read String.vi"("Name"=w302) -> ("String"=w305:string)  [unwired: 9 in, 1 out]
            n163 = Bundle("Numeric"=w304, "String"=w305) -> (→"Progress":cluster{"Numeric":dbl, "String":string})  [unwired: 1 in]
          }
          frame "" {
            n164 = property on="Progress" class="Clust (strict)"("Visible"=FALSE) -> ()  [unwired: 2 in, 2 out]
            n165 = local write "Test Name"(u16 0) -> ()
          }
        }
        n166 = call <vilib>:"Connextion Info.vi"() -> ("Connected"=→"NT Connection":bool)  [unwired: 10 in, 1 out]
      }
      event "Test Tree": Value Change {
        # "Show appropriate\ncontrols"
        n167 = event-data() -> ("CtlRef"=w314:refnum<vi>, "NewVal"=w312:string)  [unwired: 1 in]
        n168 = call <vilib>:"WPI_UtilitiesGetTreeIOName.vi"("NewVal"=w312, "TreeControl in"=w314) -> ("I/O Name"=w315:string)  [unwired: 9 in]
        n169 = case shown="\"Analog Out\", \"Motor\", \"PWM\"" w315 {
          selector: w315 -> [_ w322 _ w344 w353 _]
          tunnel: w312 -> [_ _ w341 w343 _ w360]
          tunnel: w311 -> [_ _ _ _ _ w359]
          frame Default {
            w317 = FALSE ("Visible")
            w316 = FALSE ("Visible")
            n170 = property on="Motor" class="Clust (strict)"("Visible"=w316) -> ()  [unwired: 2 in, 2 out]
            n171 = property on="Test Ring" class="Ring (strict)"("Visible"=w316) -> ()  [unwired: 2 in, 2 out]
            n172 = property on="Rev/Fwd" class="Clust (strict)"("Visible"=w317) -> ()  [unwired: 2 in, 2 out]
            n173 = property on="On/Off" class="Bool (strict)"("Visible"=w317) -> ()  [unwired: 2 in, 2 out]
            n174 = property on="Test Slider" class="Slide (strict)"("Visible"=w317) -> ()  [unwired: 2 in, 2 out]
          }
          frame "Analog Out", "Motor", "PWM" {
            w323 = FALSE ("Visible")
            n175 = case shown="\"Analog Out\"" w322 {
              tunnel: [1.0 ("Value") -1.0 ("Value") 0.0 ("Value")] -> w321
              tunnel: [255.0 ("Value") 1.0 ("Value") 5.0 ("Value")] -> w320
              tunnel: [128.0 ("Value") 0.0 ("Value") 0.0 ("Value")] -> w319
              tunnel: [64.0 ("Value") 0.5 ("Value") 1.0 ("Value")] -> w318
              frame "PWM" {
              }
              frame "Motor", Default {
              }
              frame "Analog Out" {
              }
            }
            n176 = property on="Motor" class="Clust (strict)"("Visible"=TRUE) -> ()  [unwired: 2 in, 2 out]
            n177 = property on="Value" class="Slide (strict)"("Value"=w319, "Scale.Minimum"=w321, "Scale.Maximum"=w320, "Scale.Increment"=w318) -> ()  [unwired: 2 in, 2 out]
            n178 = property on="On/Off" class="Bool (strict)"("Visible"=w323) -> ()  [unwired: 2 in, 2 out]
            n179 = property on="Test Slider" class="Slide (strict)"("Visible"=w323) -> ()  [unwired: 2 in, 2 out]
            n180 = property on="Test Ring" class="Ring (strict)"("Visible"=w323) -> ()  [unwired: 2 in, 2 out]
            n181 = property on="Rev/Fwd" class="Clust (strict)"("Visible"=w323) -> ()  [unwired: 2 in, 2 out]
          }
          frame "Servo" {
            w339 = FALSE ("Visible")
            n182 = call <vilib>:"NT Read Number.vi"("Name"=w341) -> ("Numeric"=w340:dbl)  [unwired: 9 in, 1 out]
            n183 = property on="Test Slider" class="Slide (strict)"("Visible"=TRUE, "Scale.Maximum"=170.0 ("Scale.Range:Maximum")) -> ()  [unwired: 2 in, 2 out]
            n184 = local write "Test Slider"(w340) -> ()
            n185 = property on="Motor" class="Clust (strict)"("Visible"=w339) -> ()  [unwired: 2 in, 2 out]
            n186 = property on="Rev/Fwd" class="Clust (strict)"("Visible"=w339) -> ()  [unwired: 2 in, 2 out]
            n187 = property on="On/Off" class="Bool (strict)"("Visible"=w339) -> ()  [unwired: 2 in, 2 out]
            n188 = property on="Test Ring" class="Ring (strict)"("Visible"=w339) -> ()  [unwired: 2 in, 2 out]
          }
          frame "Relay", "Solenoid" {
            w342 = FALSE ("Visible")
            n189 = property on="Motor" class="Clust (strict)"("Visible"=w342) -> ()  [unwired: 2 in, 2 out]
            n190 = property on="Test Slider" class="Slide (strict)"("Visible"=w342) -> ()  [unwired: 2 in, 2 out]
            n191 = Search and Replace String(input string=w343, search string="/Value  **", replace string="/Direction") -> (result string=w349:string)  [unwired: 5 in, 3 out]
            n192 = property on="Test Ring" class="Ring (strict)"("Visible"=w342) -> ()  [unwired: 2 in, 2 out]
            n193 = call <vilib>:"NT Read String.vi"("Name"=w349) -> ("String"=w347:string)  [unwired: 9 in, 1 out]
            n194 = Equal?(x="Both directions", y=w347) -> (x = y?=w345:bool)
            n195 = Not(x=w345) -> (.not. x?=w346:bool)
            n196 = property on="Rev/Fwd" class="Clust (strict)"("Visible"=w345) -> ()  [unwired: 2 in, 2 out]
            n197 = property on="On/Off" class="Bool (strict)"("Visible"=w346, "Caption.Text"=w344) -> ()  [unwired: 2 in, 2 out]
          }
          frame "Compressor", "Digital Out" {
            w352 = FALSE ("Visible")
            # "Get direction and finish"
            n198 = property on="Motor" class="Clust (strict)"("Visible"=w352) -> ()  [unwired: 2 in, 2 out]
            n199 = property on="Test Slider" class="Slide (strict)"("Visible"=w352) -> ()  [unwired: 2 in, 2 out]
            n200 = property on="Test Ring" class="Ring (strict)"("Visible"=w352) -> ()  [unwired: 2 in, 2 out]
            n201 = property on="On/Off" class="Bool (strict)"("Visible"=TRUE, "Caption.Text"=w353) -> ()  [unwired: 2 in, 2 out]
            n202 = property on="Rev/Fwd" class="Clust (strict)"("Visible"=FALSE) -> ()  [unwired: 2 in, 2 out]
          }
          frame "Camera" {
            n203 = call <vilib>:"Get Last Path Segment.vi"("String in"=w360) -> ("String out"=w361:string)  [unwired: 10 in]
            n204 = property on="On/Off" class="Bool (strict)"("Visible"=FALSE) -> ()  [unwired: 2 in, 2 out]
            n205 = property on="Motor" class="Clust (strict)"("Visible"=FALSE) -> ()  [unwired: 2 in, 2 out]
            n206 = property on="Rev/Fwd" class="Clust (strict)"("Visible"=FALSE) -> ()  [unwired: 2 in, 2 out]
            n207 = case shown="\"White Balance  **\"" w361 {
              tunnel: w360 -> [w367 w376 w385 w394 w403 _ w409]
              tunnel: w359 -> [w365 w373 w382 w391 w400 _ _]
              frame "Size  **" {
                n208 = Index Array(array=w365) -> (element=w364:cluster{string[]})  [unwired: 1 in]
                n209 = call <vilib>:"NT Read String.vi"("Name"=w367) -> ("String"=w366:string)  [unwired: 9 in, 1 out]
                n210 = Unbundle(w364) -> (w362:string[])
                n211 = Match First String(2:w362, 3:w366) -> (0:w363:i32)  [unwired: 1 out]
                n212 = property on="Test Ring" class="Ring (strict)"("Value"=w363, "Strings []"=w362) -> ()  [unwired: 2 in, 2 out]
                n213 = property on="Test Ring" class="Ring (strict)"("Visible"=TRUE) -> ()  [unwired: 2 in, 2 out]
                n214 = property on="Test Slider" class="Slide (strict)"("Visible"=FALSE) -> ()  [unwired: 2 in, 2 out]
              }
              frame "White Balance  **" {
                n215 = Index Array(array=w373, index=1) -> (element=w374:cluster{string[]})
                n216 = call <vilib>:"NT Read String.vi"("Name"=w376) -> ("String"=w375:string)  [unwired: 9 in, 1 out]
                n217 = Unbundle(w374) -> (w371:string[])
                n218 = Match First String(2:w371, 3:w375) -> (0:w370:i32)  [unwired: 1 out]
                n219 = property on="Test Ring" class="Ring (strict)"("Value"=w370, "Strings []"=w371) -> ()  [unwired: 2 in, 2 out]
                n220 = property on="Test Ring" class="Ring (strict)"("Visible"=TRUE) -> ()  [unwired: 2 in, 2 out]
                n221 = property on="Test Slider" class="Slide (strict)"("Visible"=FALSE) -> ()  [unwired: 2 in, 2 out]
              }
              frame "Exposure  **" {
                n222 = Index Array(array=w382, index=2) -> (element=w383:cluster{string[]})
                n223 = call <vilib>:"NT Read String.vi"("Name"=w385) -> ("String"=w384:string)  [unwired: 9 in, 1 out]
                n224 = Unbundle(w383) -> (w379:string[])
                n225 = Match First String(2:w379, 3:w384) -> (0:w380:i32)  [unwired: 1 out]
                n226 = property on="Test Ring" class="Ring (strict)"("Value"=w380, "Strings []"=w379) -> ()  [unwired: 2 in, 2 out]
                n227 = property on="Test Ring" class="Ring (strict)"("Visible"=TRUE) -> ()  [unwired: 2 in, 2 out]
                n228 = property on="Test Slider" class="Slide (strict)"("Visible"=FALSE) -> ()  [unwired: 2 in, 2 out]
              }
              frame "Exposure Priority  **" {
                n229 = Index Array(array=w391, index=3) -> (element=w392:cluster{string[]})
                n230 = call <vilib>:"NT Read String.vi"("Name"=w394) -> ("String"=w393:string)  [unwired: 9 in, 1 out]
                n231 = Unbundle(w392) -> (w388:string[])
                n232 = Match First String(2:w388, 3:w393) -> (0:w389:i32)  [unwired: 1 out]
                n233 = property on="Test Ring" class="Ring (strict)"("Value"=w389, "Strings []"=w388) -> ()  [unwired: 2 in, 2 out]
                n234 = property on="Test Ring" class="Ring (strict)"("Visible"=TRUE) -> ()  [unwired: 2 in, 2 out]
                n235 = property on="Test Slider" class="Slide (strict)"("Visible"=FALSE) -> ()  [unwired: 2 in, 2 out]
              }
              frame "Color Enable  **" {
                n236 = Index Array(array=w400, index=4) -> (element=w401:cluster{string[]})
                n237 = call <vilib>:"NT Read String.vi"("Name"=w403) -> ("String"=w402:string)  [unwired: 9 in, 1 out]
                n238 = Unbundle(w401) -> (w397:string[])
                n239 = Match First String(2:w397, 3:w402) -> (0:w398:i32)  [unwired: 1 out]
                n240 = property on="Test Ring" class="Ring (strict)"("Value"=w398, "Strings []"=w397) -> ()  [unwired: 2 in, 2 out]
                n241 = property on="Test Ring" class="Ring (strict)"("Visible"=TRUE) -> ()  [unwired: 2 in, 2 out]
                n242 = property on="Test Slider" class="Slide (strict)"("Visible"=FALSE) -> ()  [unwired: 2 in, 2 out]
              }
              frame Default {
                n243 = property on="Test Ring" class="Ring (strict)"("Visible"=FALSE) -> ()  [unwired: 2 in, 2 out]
                n244 = property on="Test Slider" class="Slide (strict)"("Visible"=FALSE) -> ()  [unwired: 2 in, 2 out]
              }
              frame "Brightness  **", "Color Level  **", "Compression  **", "FPS  **", "Sharpness  **" {
                n245 = call <vilib>:"NT Read Number.vi"("Name"=w409) -> ("Numeric"=w408:dbl)  [unwired: 9 in, 1 out]
                n246 = local write "Test Slider"(w408) -> ()
                n247 = property on="Test Slider" class="Slide (strict)"("Visible"=TRUE, "Scale.Maximum"=100.0 ("Scale.Range:Maximum")) -> ()  [unwired: 2 in, 2 out]
                n248 = property on="Test Ring" class="Ring (strict)"("Visible"=FALSE) -> ()  [unwired: 2 in, 2 out]
              }
            }
          }
        }
        n249 = property on="Progress" class="Clust (strict)"("Visible"=FALSE) -> ()  [unwired: 2 in, 2 out]
      }
      event "Test Name": Mouse Enter {
        # "Populate the ring with the list of tests"
        n250 = event-data() -> ()  [unwired: 1 in, 1 out]
        n251 = call <vilib>:"NT Read String Array.vi"("Name"="/TestMode/TestList") -> ("String Array"=w418:string[])  [unwired: 9 in, 1 out]
        n252 = Build Array (concatenate)("Select the test to run...", w418) -> (w417:string[])
        n253 = property on="Test Name" class="Ring (strict)"("Strings []"=w417) -> ()  [unwired: 2 in, 2 out]
      }
      event "Test Name": Value Change {
        w421 = FALSE ("Visible")
        # "Tell the robot the test name to run"
        n254 = event-data() -> ("NewVal"=w425:u16)  [unwired: 1 in]
        n255 = property on="Test Name" class="Ring (strict)"() -> ("Strings []"=w426:string[])  [unwired: 2 in, 2 out]
        n256 = local write "Progress"(T4 {"Test Progress"=0, "Test Progress Text"=""} ("Progress")) -> ()
        n257 = Index Array(array=w426, index=w425) -> (element=w424:string)
        n258 = call <vilib>:"NT Write String.vi"("String"=w424, "Name"="/TestMode/TestName") -> ()  [unwired: 9 in, 1 out]
        n259 = property on="Progress" class="Clust (strict)"("Visible"=TRUE) -> ()  [unwired: 2 in, 2 out]
        n260 = property on="Motor" class="Clust (strict)"("Visible"=w421) -> ()  [unwired: 2 in, 2 out]
        n261 = property on="Test Slider" class="Slide (strict)"("Visible"=w421) -> ()  [unwired: 2 in, 2 out]
        n262 = property on="On/Off" class="Bool (strict)"("Visible"=w421) -> ()  [unwired: 2 in, 2 out]
        n263 = property on="Rev/Fwd" class="Clust (strict)"("Visible"=w421) -> ()  [unwired: 2 in, 2 out]
        n264 = property on="Test Ring" class="Ring (strict)"("Visible"=w421) -> ()  [unwired: 2 in, 2 out]
      }
      event "Select Auto": Mouse Enter {
        # "Populate the combo box with the list of autonomous options"
        n265 = event-data() -> ()  [unwired: 1 in, 1 out]
        n266 = call <vilib>:"NT Read String Array.vi"("Name"="Auto List") -> ("String Array"=w428:string[])  [unwired: 9 in, 1 out]
        n267 = property on="Select Auto" class="CmbBox"("Strings[]"=w428) -> ()  [unwired: 2 in, 2 out]
      }
      event "Select Auto": Value Change {
        # "User modified the Auto Selection. Write to NT variable so robot knows."
        n268 = event-data() -> ("NewVal"=w432:string)  [unwired: 1 in]
        n269 = call <vilib>:"NT Write String.vi"("String"=w432, "Name"="Auto Selector") -> ()  [unwired: 9 in, 1 out]
      }
      event "Command Selection": Value Change {
        # "Get the params and show in table"
        n270 = event-data() -> ("NewVal"=w439:i32)  [unwired: 1 in]
        n271 = property on="Command Selection" class="MCListbox (strict)"() -> ("ItemNames"=w437:string[][])  [unwired: 2 in, 2 out]
        n272 = call <vilib>:"WPI_DashboardUpdate Command Params.vi"("NewVal"=w439, "Commands"=w437, "Param Tbl"=w438) -> ()  [unwired: 8 in, 1 out]
      }
      event "Execute Command": Value Change {
        # "Started one, Unique ID holds\nresponse"
        n273 = event-data() -> ()  [unwired: 1 in, 1 out]
        n274 = property on="Command Selection" class="MCListbox (strict)"() -> ("ItemNames"=w451:string[][])  [unwired: 2 in, 2 out]
        n275 = Index Array(array=w451, index (row)="Command Selection", index (col)=0) -> (element=w449:string)
        n276 = call <vilib>:"Invoke Commands.vi"("Command Params"="Command Params", "Function Name"=w449) -> ("Params"=w445:u8, "Started"=w444:bool)  [unwired: 7 in, 1 out]
        n277 = Array Subset(array="Command Params", length (row)=w445) -> (w446:string[][])  [unwired: 3 in]
        n278 = Select(t="Executing" ("Cmd Status"), s=w444, f="" ("Cmd Status")) -> (s? t:f=→"Cmd Status":string)
      }
      event "Command Selection": Double Click {
        n279 = event-data() -> ("Row"=w461:i32)  [unwired: 1 in]
        n280 = property on="Command Selection" class="MCListbox (strict)"() -> ("ItemNames"=w464:string[][])  [unwired: 2 in, 2 out]
        n281 = local read "Command Params"() -> (w459:string[][])
        n282 = Index Array(array=w464, index (row)=w461, index (col)=0) -> (element=w462:string)
        n283 = call <vilib>:"Invoke Commands.vi"("Command Params"=w459, "Function Name"=w462) -> ("Params"=w458:u8, "Started"=w453:bool)  [unwired: 7 in, 1 out]
        n284 = Array Subset(array=w459, length (row)=w458) -> (w457:string[][])  [unwired: 3 in]
        n285 = Select(t="Executing" ("Cmd Status"), s=w453, f="" ("Cmd Status")) -> (s? t:f=w454:string)
        n286 = local write "Cmd Status"(w454) -> ()
      }
      event "CheckList": Double Click {
        # "Shift clears all"
        # "Update symbols on the listbox"
        n287 = event-data() -> ("PlatMods.Shift"=w467:bool, "Row"=w469:i32)  [unwired: 1 in]
        n288 = case shown="True" w467 {
          tunnel: w469 -> [w473 _]
          tunnel: 1 -> [w472 _]
          frame False {
            n289 = property on="CheckList" class="LstBox (strict)"() -> ("Item Symbols"=w471:i32[])  [unwired: 2 in, 2 out]
            n290 = Replace Array Subset(array=w471, new element=w472, index=w473) -> (w470:i32[])
            n291 = property on="CheckList" class="LstBox (strict)"("Item Symbols"=w470) -> ()  [unwired: 2 in, 2 out]
          }
          frame True {
            w474 = 0 ("Top Row")
            n292 = property on="CheckList" class="LstBox (strict)"() -> ("Number of Rows"=w476:u32)  [unwired: 2 in, 2 out]
            n293 = Initialize Array(0, w476) -> (w475:i32[])
            n294 = property on="CheckList" class="LstBox (strict)"("Top Row"=w474, "Value"=w474, "Item Symbols"=w475) -> ()  [unwired: 2 in, 2 out]
          }
        }
      }
      event "CheckList": Key Down {
        # "Update symbols on the listbox\nLeft and right keys check and uncheck"
        n295 = event-data() -> ("VKey"=w481:T16)  [unwired: 1 in]
        n296 = case shown="\"Left\", \"Right\"" w481 {
          selector: w481 -> [w486 _]
          tunnel: eventvkey."Left" ("VKey") -> [w484 _]
          frame "Left", "Right" {
            n297 = Equal?(x=w484, y=w486) -> (x = y?=w485:bool)
            n298 = Select(t=0, s=w485, f=1) -> (s? t:f=w487:i32)
            n299 = property on="CheckList" class="LstBox (strict)"() -> ("Item Symbols"=w490:i32[])  [unwired: 2 in, 2 out]
            n300 = Replace Array Subset(array=w490, new element=w487, index="CheckList") -> (w489:i32[])
            n301 = property on="CheckList" class="LstBox (strict)"("Item Symbols"=w489) -> ()  [unwired: 2 in, 2 out]
          }
          frame Default {
          }
        }
      }
      event "DB Camera Config": Value Change {
        # "Show or hide the cluster of controls, store in ini file"
        n302 = event-data() -> ("NewVal"=w495:bool)  [unwired: 1 in]
        n303 = case shown="False" w495 {
          tunnel: w494 -> [w504 _]
          tunnel: [w497 w515] -> w493
          tunnel: w492 -> [w496 w515]
          frame False {
            w511 = "Camera"
            w514 = FALSE ("Visible")
            n304 = local read "Camera Settings"() -> (w503:T2)
            n305 = Index Array(array=w504) -> (element=w507:cluster{string[]})  [unwired: 1 in]
            n306 = Unbundle(w503) -> ("Frame Rate"=w502:i32, "Compression"=w501:i32, "Size"=w505:u16)
            n307 = Unbundle(w507) -> (w506:string[])
            n308 = Index Array(array=w506, index=w505) -> (element=w500:string)
            n309 = call-poly <vilib>:"Write Key.vi"("section"=w511, "value"=w500, "key"="Size", "refnum"=w496) -> ("refnum out"=w513:T14)  [unwired: 2 in, 5 out]
            n310 = call-poly <vilib>:"Write Key.vi"("section"=w511, "value"=w502, "key"="FrameRate", "refnum"=w513) -> ("refnum out"=w512:T14)  [unwired: 1 in, 6 out]
            n311 = property on="Camera Settings" class="Clust (strict)"("Visible"=w514) -> ()  [unwired: 2 in, 2 out]
            n312 = local write "DB Camera Config"(w514) -> ()
            n313 = call-poly <vilib>:"Write Key.vi"("section"=w511, "value"=w501, "key"="Compression", "refnum"=w512) -> ("refnum out"=w498:T14)  [unwired: 1 in, 6 out]
            n314 = call <vilib>:"Close Config Data.vi"("refnum"=w498) -> ("file path"=w499:path)  [unwired: 2 in, 8 out]
            n315 = call <vilib>:"Open Config Data.vi"("configuration file path"=w499) -> ("refnum"=w497:T14)  [unwired: 8 in, 2 out]
          }
          frame True {
            n316 = property on="Camera Settings" class="Clust (strict)"("Visible"=TRUE) -> ()  [unwired: 2 in, 2 out]
          }
        }
      }
      event "Camera Settings": Value Change {
        # "Update summary string when any elements of DB camera change"
        n317 = event-data() -> ("NewVal"=w529:T2)  [unwired: 1 in]
        n318 = Index Array(array=w525) -> (element=w524:cluster{string[]})  [unwired: 1 in]
        n319 = Unbundle(w529) -> ("Frame Rate"=w520:i32, "Compression"=w519:i32, "Size"=w522:u16)
        n320 = Unbundle(w524) -> (w523:string[])
        n321 = Index Array(array=w523, index=w522) -> (element=w521:string)
        n322 = Format Into String(format string="%s   %dfps   %d%%", w521, w520, w519) -> (resulting string=w526:string)  [unwired: 2 in, 1 out]
        n323 = Build Array(w526) -> (w527:string[])
        n324 = property on="DB Camera Config" class="Bool (strict)"("Strings [4]"=w527) -> ()  [unwired: 2 in, 2 out]
      }
      event "Motor.Enable": Value Change {
        # "When the test mode otor enable helper is set, update that\ntree row item's value"
        n325 = event-data() -> ("NewVal"=w536:bool)  [unwired: 1 in]
        n326 = Unbundle("Motor") -> ("Value"=w535:dbl)  [unwired: 1 out]
        n327 = Select(t=w535, s=w536, f=0.0) -> (s? t:f=w533:dbl)
        n328 = call <vilib>:"NT Write Number.vi"("Numeric"=w533, "Name"=w532) -> ()  [unwired: 9 in, 1 out]
      }
      event "Test Slider": Value Change {
        # "When the test mode slider helper is set, update that\ntree row item's value"
        n329 = event-data() -> ("NewVal"=w540:dbl)  [unwired: 1 in]
        n330 = call <vilib>:"NT Write Number.vi"("Numeric"=w540, "Name"=w541) -> ()  [unwired: 9 in, 1 out]
      }
      event "On/Off": Value Change {
        # "When the test mode on/off helper value is set, update that\ntree row item's value"
        n331 = event-data() -> ("NewVal"=w546:bool)  [unwired: 1 in]
        n332 = Boolean To (0,1)(Boolean=w546) -> (0, 1=w545:i16)
        n333 = call <vilib>:"NT Write Number.vi"("Numeric"=w545, "Name"=w544) -> ()  [unwired: 9 in, 1 out]
      }
      event "Rev/Fwd": Value Change {
        # "When the test mode helper value for relays is set, update that\ntree row item's value"
        n334 = event-data() -> ("NewVal.Forward"=w555:bool, "NewVal.Reverse"=w554:bool)  [unwired: 1 in]
        n335 = Boolean To (0,1)(Boolean=w555) -> (0, 1=w551:i16)
        n336 = Boolean To (0,1)(Boolean=w554) -> (0, 1=w553:i16)
        n337 = Negate(x=w553) -> (-x=w552:i16)
        n338 = Add(x=w551, y=w552) -> (x+y=w550:i16)
        n339 = call <vilib>:"NT Write Number.vi"("Numeric"=w550, "Name"=w549) -> ()  [unwired: 9 in, 1 out]
      }
      event "Test Ring": Value Change {
        # "When a test mode helper value is selected from the ring,\nset the tree item's variable to the string value"
        n340 = event-data() -> ("NewVal"=w560:u16)  [unwired: 1 in]
        n341 = property on="Test Ring" class="Ring (strict)"() -> ("Strings []"=w561:string[])  [unwired: 2 in, 2 out]
        n342 = Index Array(array=w561, index=w560) -> (element=w559:string)
        n343 = call <vilib>:"NT Write String.vi"("String"=w559, "Name"=w558) -> ()  [unwired: 9 in, 1 out]
      }
      event "Rec Mode": Value Change {
        # "Update globals for recording mode and path to read log from.\nClear when logging and let NetworkTables set path for vision to\nuse."
        n344 = event-data() -> ("NewVal"=w573:enum32{"Stop", "Record", "Playback"})  [unwired: 1 in]
        n345 = global write "WPI_DashboardLogging Global.vi" "Logging Filename"(path "") -> ()
        n346 = global write "WPI_DashboardLogging Global.vi" "Recording"(w573) -> ()
        n347 = case shown="\"Playback\"" w573 {
          tunnel: w572 -> [_ w575 w584]
          tunnel: [_ _ w583] -> w569
          tunnel: [_ _ w582] -> _
          tunnel: w567 -> [_ _ w580]
          tunnel: cluster{i32, i32} {-250, 170} -> [_ _ w579]
          tunnel: [_ _ T17 {"Image Size"=TRUE, "Image Type"=TRUE, "Pixel Value"=TRUE, "ROI Information"=TRUE, "Zoom Factor"=FALSE} ("Image Information Shown:All Elements")] -> w565
          tunnel: [_ _ TRUE ("Zoom Factor")] -> w564
          tunnel: w563 -> [_ _ w576]
          frame Default {
          }
          frame "Stop", "Record" {
            # "Place Window too"
            n348 = invoke class="VI" method="FP.Close"(reference=w575) -> (reference out=w574:refnum<vi>)  [unwired: 2 in, 2 out]
            n349 = invoke class="VI" method="Abort VI"(reference=w574) -> ()  [unwired: 2 in, 3 out]
          }
          frame "Playback" {
            n350 = call "Open Playback Panel.vi"("Offset"=w579, "DB VI Ref"=w580, "Playback in"=w584) -> ("Playback out"=w581:refnum<vi>)  [unwired: 8 in]
            n351 = register-events(w581, w576) -> (reference out=w583:refnum<event-registration>, error out=w582:errorcluster)  [unwired: 2 in]
          }
        }
        n352 = property on="Camera Image" class="ImageControl"("Image Information Shown"=w565, "Image Information Visible"=w564) -> ()  [unwired: 2 in, 2 out]
        n353 = call <vilib>:"WPI_DashboardNT Log FieldName Cache.vi"("Operation"=enum16{"Lookup/Add", "Index", "Clear"}."Clear") -> ()  [unwired: 8 in, 3 out]
      }
      event Panel Close {
        w586 = enum32{"Stop", "Record", "Playback"}."Stop" ("Rec Mode")
        # "Playback window has been closed, abort"
        n354 = event-data() -> ()  [unwired: 1 in, 4 out]
        n355 = local write "Rec Mode"(w586) -> ()
        n356 = global write "WPI_DashboardLogging Global.vi" "Recording"(w586) -> ()
      }
      event Panel Close {
        # "Abort playback window and ourself"
        n357 = event-data() -> ()  [unwired: 1 in, 4 out]
        n358 = invoke class="VI" method="FP.Close"(reference=w592) -> (reference out=w591:refnum<vi>)  [unwired: 2 in, 2 out]
        n359 = invoke class="VI" method="Abort VI"(reference=w591) -> (error out=w590:errorcluster)  [unwired: 2 in, 2 out]
        n360 = invoke class="VI" method="Abort VI"(error in=w590) -> ()  [unwired: 2 in, 3 out]
      }
      event User Event {
        n361 = event-data() -> ("IDs"=w600:cluster{"RPC field ID":u16, "Unique ID":u16}, "String"=w599:string)  [unwired: 1 in]
        n362 = Bundle("IDs"=w600, "String"=w599) -> (w598:T6)  [unwired: 1 in]
        n363 = call <vilib>:"Retrieve RPC Response.vi"("RPC Response"=w598) -> ("Output"=w595:string[][])  [unwired: 10 in]
        n364 = Build Array (concatenate)(w593, w595) -> (w594:string[][])
        n365 = local write "Command Params"(w594) -> ()
        n366 = local write "Cmd Status"("" ("Cmd Status")) -> ()
      }
      event "Vision": Value Change {
        # "Enable/Disable Compression slider.\nHW USB is hard-coded into the camera"
        n367 = event-data() -> ("NewVal"=w607:u16)  [unwired: 1 in]
        n368 = Equal?(x=w607, y=u32 2 ("milliseconds to wait")) -> (x = y?=w605:bool)
        n369 = Select(t=T18."Disabled and Grayed Out" ("Disabled"), s=w605, f=T18."Enabled" ("Disabled")) -> (s? t:f=w602:T18)
        n370 = property on="Compression" class="Slide (strict)"("DisabledEnum"=w602) -> ()  [unwired: 2 in, 2 out]
      }
      event "Tree": Double Click {
        n371 = event-data() -> ("PlatMods"=w612:T21, "Tag"=w611:string)  [unwired: 1 in]
        n372 = Unbundle(w612) -> ("Shift"=w610:bool)  [unwired: 4 out]
        n373 = Not(x=w610) -> (.not. x?=w609:bool)
        n374 = call <vilib>:"NT Update Persistence.vi"("Persistence"=w609, "Name"=w611) -> ()  [unwired: 9 in, 1 out]
      }
    }
  }
  n375 = while {
    tunnel: w48 -> [w616]
    i -> [w619]
    stop <- FALSE stop-if-true
    n376 = Wait (ms)(milliseconds to wait=u32 100) -> ()  [unwired: 1 out]
    n377 = case shown="\"Playback\"" "Rec Mode" {
      tunnel: w619 -> [_ _ w634]
      tunnel: [u32 2829099 ("Base Color") u32 11141120 ("Target Color") w623] -> w615
      frame "Stop", Default {
        # "Reset the color, extra updates don't cost much"
      }
      frame "Record" {
      }
      frame "Playback" {
        # "Playback"
        n378 = Quotient & Remainder(x=w634, y=u32 50 ("milliseconds to wait")) -> (x-y*floor(x/y)=w630:u32)  [unwired: 1 out]
        n379 = Divide(x=w630, y=u32 50 ("milliseconds to wait")) -> (x/y=w627:dbl)
        n380 = Multiply(x=6.283185307179586, y=w627) -> (x*y=w632:dbl)
        n381 = Sine(x=w632) -> (sin(x)=w631:dbl)
        n382 = Absolute Value(x=w631) -> (abs(x)=w624:dbl)
        n383 = call "Interpolate RGB Color.vi"("Proportion"=w624, "Target Color"=u32 30976, "Base Color"=u32 2829099) -> ("Result Color"=w623:u32)  [unwired: 8 in]
      }
    }
    n384 = property class="Pane"(reference=w616, "PaneColor"=w615) -> ()  [unwired: 1 in, 2 out]
  }
  n385 = local write "Dashboard Tab"(T1."Drive" ("Dashboard Tab")) -> ()
  n386 = property on="On/Off" class="Bool (strict)"("Visible"=w16) -> ()  [unwired: 2 in, 2 out]
  n387 = property on="Motor" class="Clust (strict)"("Visible"=w16) -> ()  [unwired: 2 in, 2 out]
  n388 = property on="Progress" class="Clust (strict)"("Visible"=w16) -> ()  [unwired: 2 in, 2 out]
  n389 = property on="Test Ring" class="Ring (strict)"("Visible"=w16) -> ()  [unwired: 2 in, 2 out]
  n390 = property on="Rev/Fwd" class="Clust (strict)"("Visible"=w16) -> ()  [unwired: 2 in, 2 out]
  n391 = property on="Camera Settings" class="Clust (strict)"("Visible"=w16) -> ()  [unwired: 2 in, 2 out]
  n392 = while {
    tunnel: u16 1741 ("timeout ms (25000)") -> [w636]
    stop <- FALSE stop-if-true
    n393 = TCP Create Listener(10:w636) -> (0:w635:errorcluster, 3:w637:refnum<k5>)  [unwired: 4 in, 1 out]
    n394 = case shown="No Error" w635 {
      selector: w635 -> [w639 _]
      tunnel: w637 -> [w640 _]
      frame No Error {
        n395 = while {
          tunnel: w640 -> [w643]
          tunnel: w639 -> [w642]
          stop <- FALSE stop-if-true
          n396 = TCP Wait On Listener(8:w642, 11:w643) -> (0:w644:errorcluster, 4:w645:refnum<k5>)  [unwired: 2 in, 3 out]
          n397 = local write "TCP"(w645) -> ()
          n398 = case shown="No Error" w644 {
            frame No Error {
            }
            frame Error {
              n399 = Wait (ms)(milliseconds to wait=u32 1000) -> ()  [unwired: 1 out]
            }
          }
        }
      }
      frame Error {
        n400 = Wait (ms)(milliseconds to wait=u32 1000) -> ()  [unwired: 1 out]
      }
    }
  }
  n401 = local write "DB Camera Config"(w16) -> ()
  n402 = local write "Command Params"(string[][] [] ("Command Params")) -> ()
  n403 = global write "WPI_DashboardLogging Global.vi" "Recording"(w42) -> ()
  n404 = local write "Command Selection"(u16 0 ("milliseconds to wait")) -> ()
  n405 = local write "Rec Mode"(w42) -> ()
